vi "Global Variables.vi"() -> ()   [LabVIEW 2016]
panel:
  in  "Calib Params?":bool
  in  "Groove?":bool
  out "Scan Count":u64
  in  "Gen Finished":bool
  out "DH Params":cluster{"d_DH":dbl[][], "ty":dbl[][]}
  in  "Section Finished?":bool
  in  "Tracking Mode":u16(ring) items=["Joint Mode", "XYZ Mode"]
  out "Tip out Posit":dbl[](array[numeric]) format="%#.3f"
  in  "Tool Offset":dbl=-50.68
  in  "us cmd":sgl min=0 max=100 step=10
  out "L5 out Posit":dbl
  out "L1 to L4 M/S cmd":dbl[](array[numeric])
  out "L5 M/S cmd":dbl
  out "elapsed time":u16
  out "file path":path
  in  "file exists?":bool
  out "zIris":dbl[](array[numeric])
  out "yIris":dbl[](array[numeric])
  out "xIris":dbl[](array[numeric])
  in  "IOP Ctrl Engaged?":bool
  out "zTraj":dbl[](array[numeric])
  out "yTraj":dbl[](array[numeric])
  out "xTraj":dbl[](array[numeric])
  out "zPC":dbl[](array[numeric])
  out "yPC":dbl[](array[numeric])
  out "xPC":dbl[](array[numeric])
  out "zACh":dbl[](array[numeric])
  out "yACh":dbl[](array[numeric])
  out "xACh":dbl[](array[numeric])
  in  "Update Traj":bool
  in  "Enforce Homing":bool
  in  "Inside RCM":bool
  out "Receive Count":u64
  out "Send Count":u64
  out "Robot Home Status":bool[](array[boolean])
  out "Robot Status Array":bool[](array[boolean])
  in  "armID":i32(ring)=1 items=["Left Arm", "Right Arm"]
  in  "armOnOff":bool
  in  "octDir":bool
  out "cyber iter. no.":u16
  out "depth counts":u16
  in  "vac digit cmd":i8
  in  "pause":bool
  out "L1 to L3 M/S cmd":dbl[](array[numeric])
  out "seconds of data":sgl
  in  "take IOP data":bool
  out "pressure sensors":sgl[](array[numeric])
  out "L4 M/S cmd":dbl
  in  "vac PID gains":cluster{"Kp":dbl, "Kd":dbl, "Ki":dbl, "Ts":dbl}={"Kp"=1.25, "Kd"=0.0, "Ki"=30.0, "Ts"=0.01}
  out "target IOP":sgl
  in  "vac PID on/off":bool
  out "L1 to L4 ctrl volt":dbl[](array[numeric])
  out "L1 to L4 robot config":dbl[](array[numeric])
  in  "plotting finished":bool
  in  "ref cluster":T1
  out "current iter. no.":u16
  out "ILC state flags":bool[](array[boolean])
  out "vac cmd":sgl
  out "reroute hold [sec]":dbl
  out "reroute transit vacf":dbl
  out "tracking timer":i32
  in  "go to regulation":bool
  out "min PC gap":dbl
  out "min AC gap":dbl
  out "AC z displacement":dbl
  out "PC z displacement":dbl
  in  "increment ctrl":dbl[](array[numeric])=[0.001, 0.005, 0.001]
  out "speed schedule":dbl
  in  "irrigate":bool
  out "last loop index":i32
  out "refractive index":dbl=1.35
  in  "joint limits":dbl[][](array[numeric])=[[-10.0, 35.0], [-35.0, 35.0], [0.1, 10.0], [-40.0, 40.0]]
  in  "assign pt out of bound":bool
  out "z monitor":dbl
  out "assign pt (x,y,z)":dbl[](array[numeric])
  in  "lock robot":bool
  out "OCT Z init Posit":dbl
  out "z rot axis":dbl
  out "z dist thld":dbl[](array[numeric])
  out "vac extremum":dbl[](array[numeric])
  in  "current run no.":u8
  in  "go to assign pt":bool
  in  "speed override":u16(ring) items=["1x", "0.5x", "0.2x", "0.1x", "PAUSE"]
  out "deform array":dbl[](array[numeric])
  in  "reset joystick":bool
  out "remote ctrl source":u16
  out "vacuum slide":i8
  out "max limit [mmHg]":dbl
  out "finished late counts":u16
  out "Accurus cluster":T2
  in  "L3 go home":bool
  out "OCT Z out Posit":dbl
  out "OCT Z cmd Posit":dbl
  out "Stage cmd Posit":dbl[](array[numeric])
  out "L1 to L4 cmd Posit":dbl[](array[numeric])
  out "L1 to L4 out Posit":dbl[](array[numeric])
  out "Stage out Posit":dbl[](array[numeric])
  in  "stop accurus":bool
  in  "state changing":bool
  out "state flag array":bool[](array[boolean])
  in  "program stop":bool
  # "0 homing finished"
  # "1 M/S initialization finished"
  # "2 trajecoty loading finished"
  # "3 aiming finished"
  # "4 insertion finished"
  # "5 tracking initialization finished"
  # "6 in tracking"
  # "7 rerouting finished"
  # "8 in regulation"
  # "0 homing finished"
  # "1 initialization finished"
  # "2 cyber learning finished"
  # "3 tracking finished"
  # "4 physical learning finished"
  # "IRISS V2"
  # "Arm"
  # "Tool"
  # "XYZ Stage"
  # "ROBOT_HARDWARE_NOT_PRESENT"
  # "ROBOT_HARDWARE_NOT_FOUND_ALL_DRIVES"
  # "ROBOT_HARDWARE_SENSOR_FAULT"
  # "ROBOT_NOT_RUNNING"
  # "ROBOT_COMMUNICATION_ERROR"
  # "ROBOT_KINEMATICS_NO_SOLUTION"
  # "ROBOT_KINEMATICS_INSERTION_LENGTH_TOO_SMALL"
  # "ROBOT_COMMAND_BEYOND_JOINT_RANGE"
  # "ROBOT_COMMAND_TOO_LARGE"
  # "button 1"
  # "button 2"
  # "button 3"
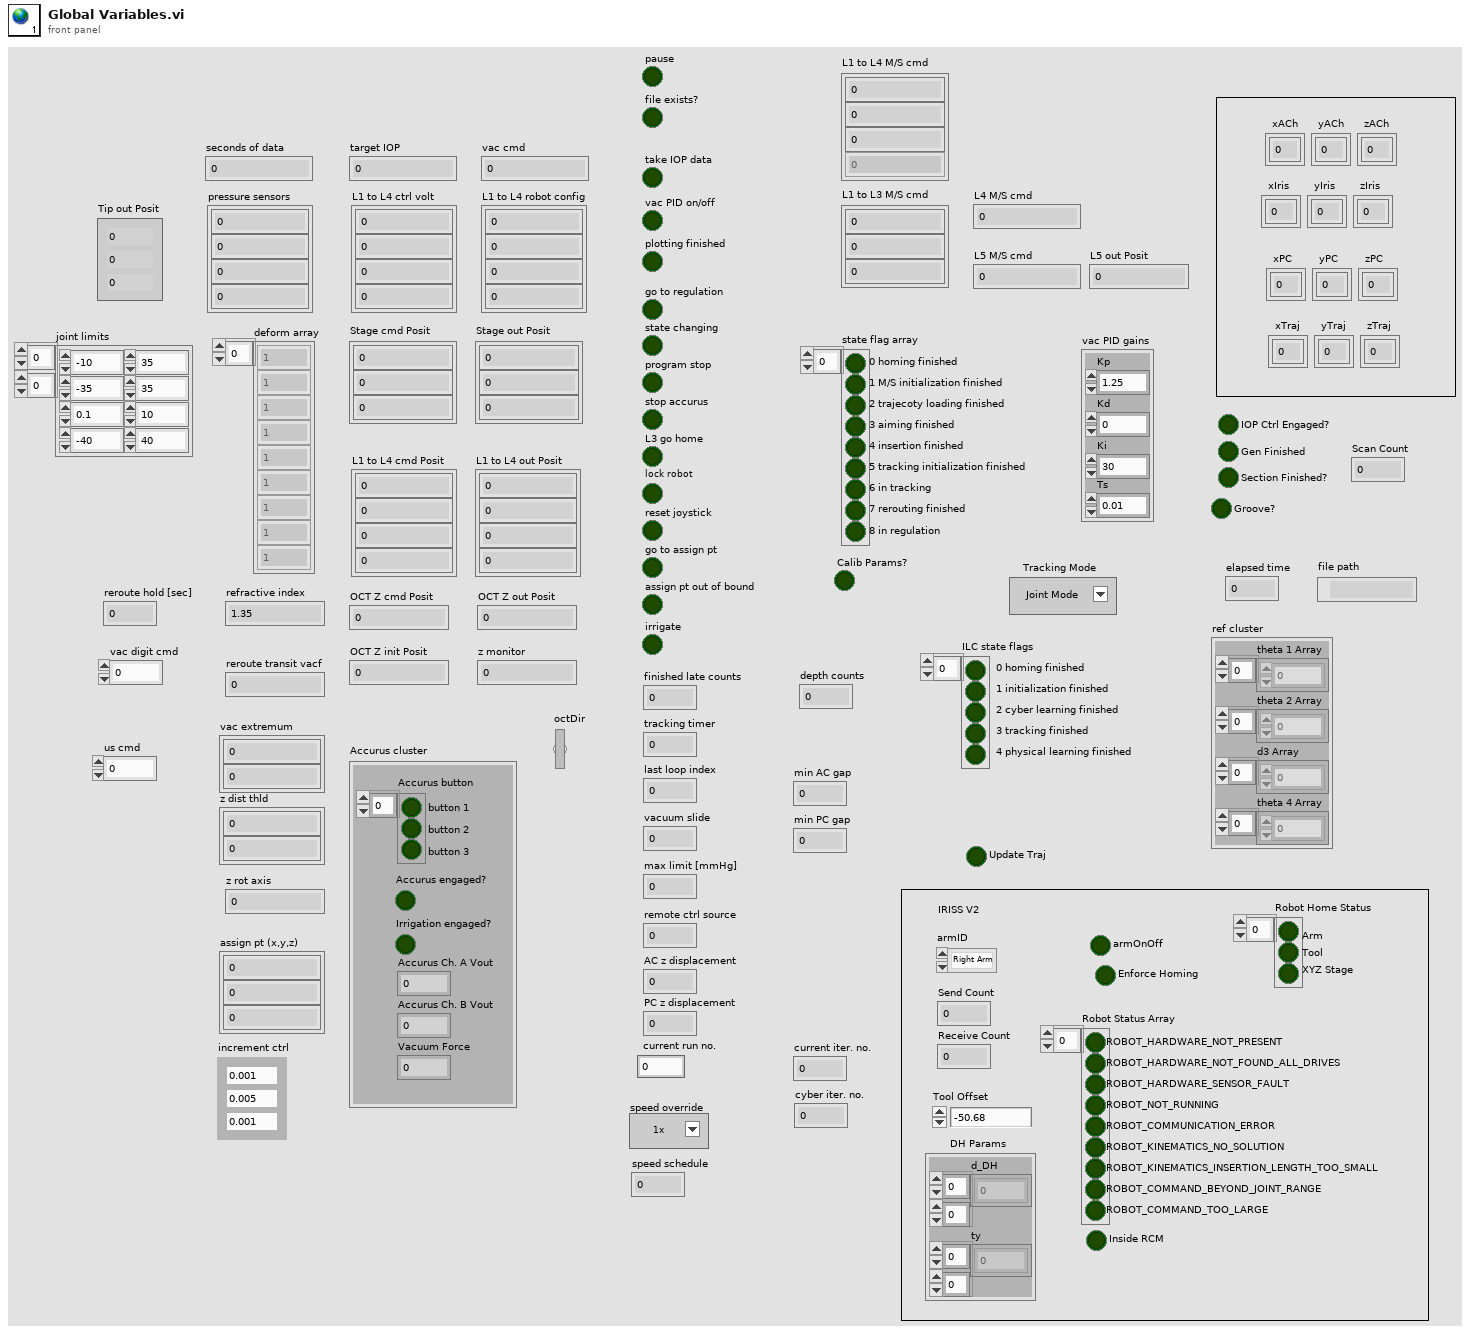
[diagram p1: front panel]
types:
  T1 = cluster{"theta 1 Array":dbl[], "theta 2 Array":dbl[], "d3 Array":dbl[], "theta 4 Array":dbl[]}
  T2 = cluster{"Accurus button":bool[], "Accurus engaged?":bool, "Vacuum Force":i32, "Accurus Ch. A Vout":dbl, "Accurus Ch. B Vout":dbl, "Irrigation engaged?":bool}
diagram:
